vi "rspvtd_Connection Notify.vi"(8 "error in":errorcluster, 11 "Data in":variant) -> (0 "error out":errorcluster, 3 "Data out":T1)   [LabVIEW 2017, in "_TCP Client.lvlib" / "TCP Client.lvclass"]
doc: "This VI converts variant data contained in the associated <b>Public API Response</b> message to its correct data type.\n---"
uses:
  TCP Client.lvclass
  rsp_Connection Notify.ctl
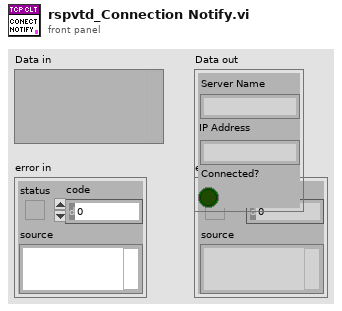
[diagram p1: front panel]
types:
  T1 = typedef "_TCP Client.lvlib/TCP Client.lvclass/rsp_Connection Notify.ctl" = cluster{"Server Name":string, "IP Address":string, "Connected?":bool}
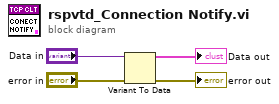
[diagram p0: block diagram]
diagram:
  n1 = Variant To Data(error in="error in", Variant="Data in") -> (data=→"Data out":T1, error out=→"error out":errorcluster)  [unwired: 1 in]
